vi "適應性控制_輸入權重係數模式(實際控制).vi"() -> ()   [LabVIEW 2010]
panel:
  in  "權重函數向量":dbl[](array[numeric])
  out "while平均時間(ms)":dbl
  out "當下ERR":dbl
  in  "number of samples":i32=100
  in  "rate":dbl=1000.0
  out "收斂時間(s)":dbl
  out "收斂燈":bool
  in  "ERR誤差低於多少V亮燈":dbl=0.05
  out "ERR message":string=" INSTRUCTIONS:\r\rNormal Use:  When using subVIs that incorporate the error in/error out (or error I/O) structure, place this handler where you want to inform the user of an error, typically at the end of the I/O data path, as the last action of the program.  If the error in error? is ERROR, the handler creates a message describing the error and its source.  If the type of dialog = 1 (default), the message is displayed to the user, who can only acknowedge it.  If the type = 2, the user can acknowledge the message or abort execution; aborting a program with active I/O is not recommended.  If the type = 0, no message is displayed; this is used to process the error programmatically, and the error out cluster elements are wired to individual terminals for that reason.  \r\rOther Use:\n\r\nlocal testing.  To test the error code of a subVI or function that does not have the error I/O structure, you can wire its error code and a source string to the local error code and error source inputs.  If error in error? indicates no error and error code is not equal to 0, the local code and source are substituted for the error in values, and error? is set TRUE (ERROR)."
  out "理想系統與FIR輸出":cluster{dbl, dbl, dbl}(graph)
  out "system輸出":dbl
  out "input_x(t)":dbl(graph)
  in  "order":i32=8
  out "FIR輸出":dbl
  in  "Stop Button":bool
  # "A0:模擬輸入 pulse_output 2"
  # "A1:理想系統 pulse_output 1"
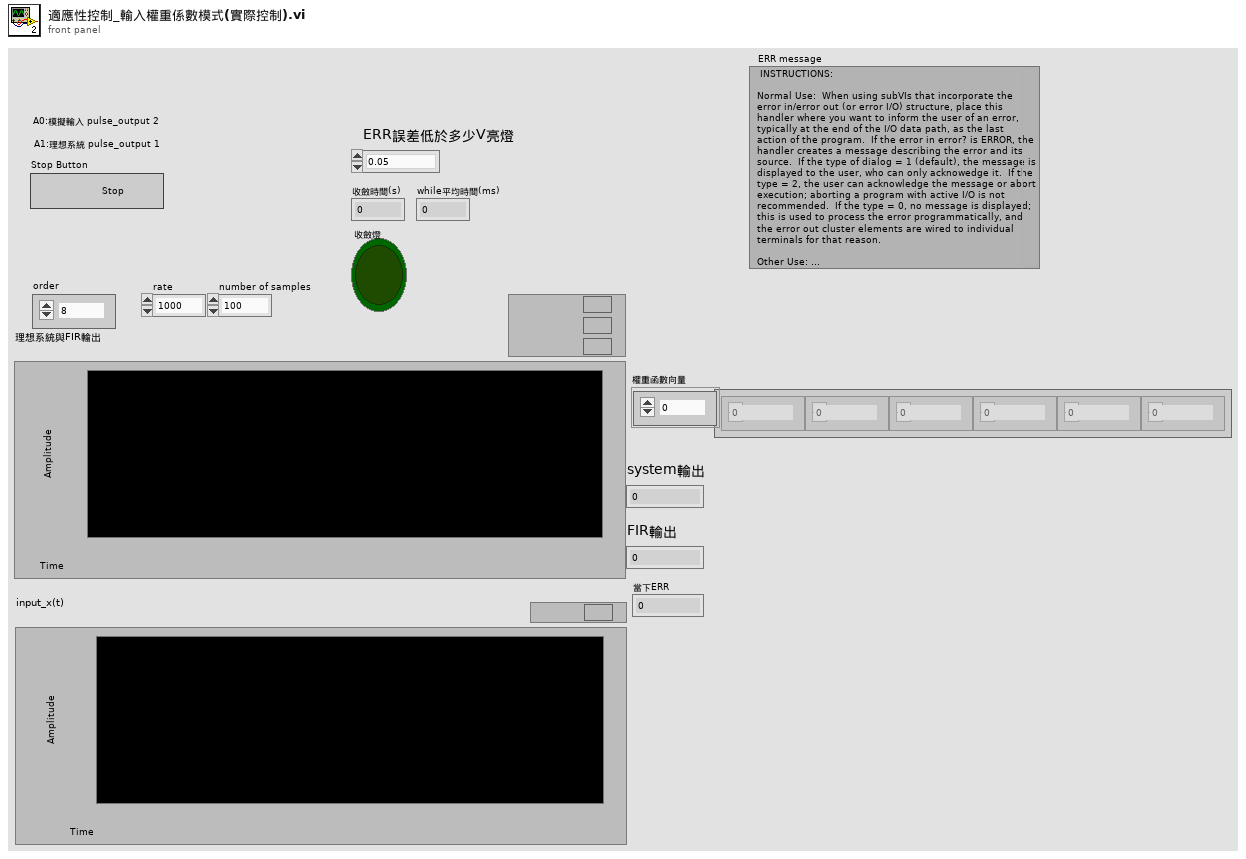
[diagram p1: front panel]
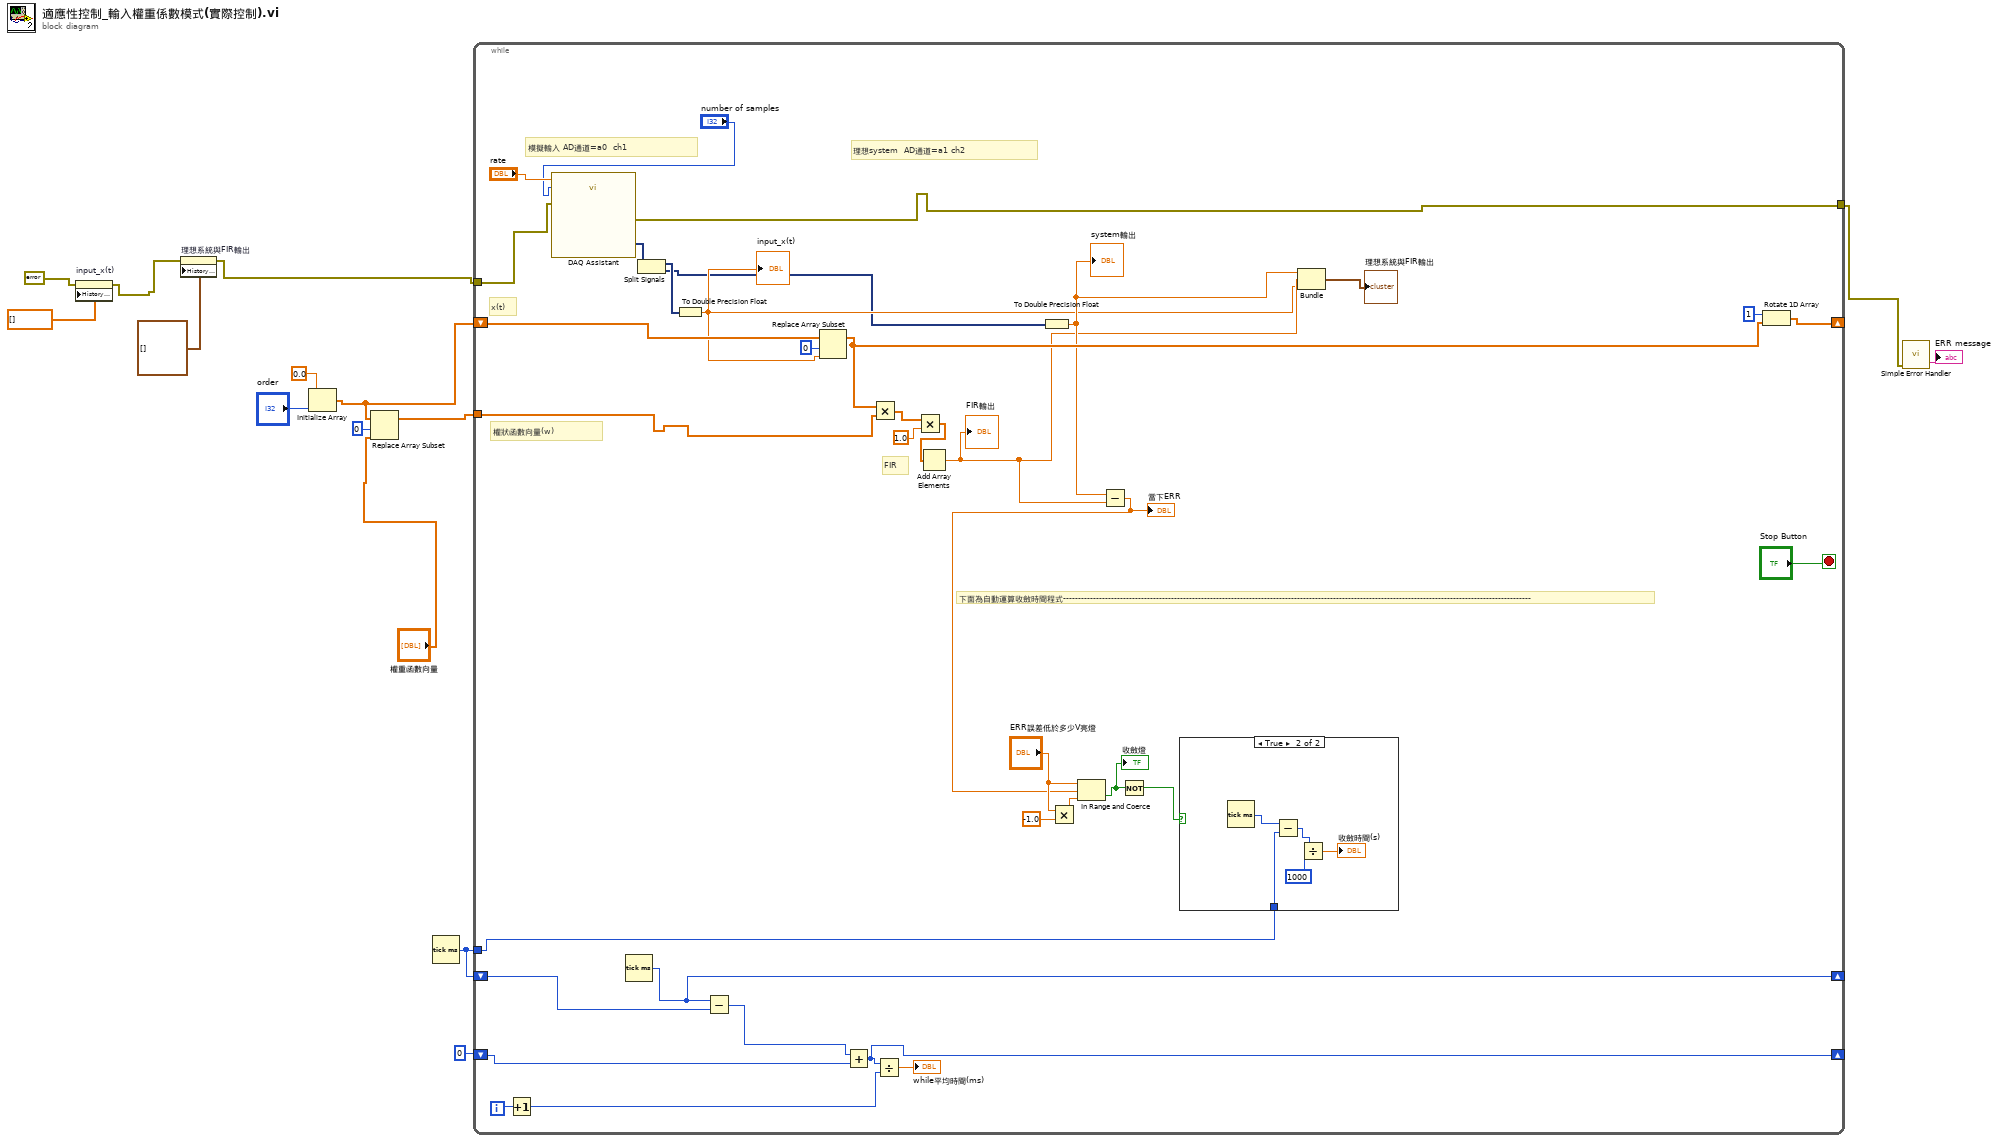
[diagram p0: block diagram]
diagram:
  n1 = property on="input_x(t)" class="WFChart (strict)"(error in=errorcluster {"status"=FALSE, "code"=0, "source"=""} ("error constant"), "History Data"=dbl[] []) -> (error out=w11:errorcluster)  [unwired: 1 in, 1 out]
  n2 = property on="理想系統與FIR輸出" class="WFChart (strict)"(error in=w11, "History Data"=cluster{dbl, dbl, dbl}[] []) -> (error out=w5:errorcluster)  [unwired: 1 in, 1 out]
  n3 = Initialize Array "Initialize Array"(0.0 ("element"), "order") -> (w7:dbl[])
  n4 = Replace Array Subset(array=w7, new element="權重函數向量", index=0) -> (w4:dbl[])
  n5 = Tick Count (ms)() -> (millisecond timer value=w8:u32)
  n6 = while {
    shift-right: [w46] -> _
    shift-left: w7 -> [w45]
    tunnel: w5 -> [w42]
    tunnel: [w17] -> w10
    shift-right: [w32] -> _
    shift-left: w8 -> [w34]
    tunnel: w8 -> [w33]
    tunnel: w4 -> [w16]
    shift-right: [w21] -> _
    shift-left: u32 0 ("y") -> [w26]
    i -> [w24]
    stop <- "Stop Button" stop-if-true
    # "下面為自動運算收斂時間程式------------------------------------------------------------------------------------------------------------------------------------------------------------"
    # "FIR"
    # "模擬輸入 AD通道=a0  ch1"
    # "權狀函數向量(w)"
    # "x(t)"
    # "理想system  AD通道=a1 ch2"
    n7 = Increment(x=w24) -> (x+1=w23:i32)
    n8 = call "DAQ Assistant"("rate"="rate", "number of samples"="number of samples", "error in"=w42) -> ("data"=w20:dynamicdata, "error out"=w17:errorcluster)  [unwired: 13 in, 2 out]
    n9 = Tick Count (ms)() -> (millisecond timer value=w32:u32)
    n10 = Split Signals(w20) -> (w19:dynamicdata, w18:dynamicdata)  [unwired: 2 in]
    n11 = To Double Precision Float(number=w19) -> (double precision float=w27:dbl)
    "input_x(t)" <- w27
    n12 = Subtract(x=w32, y=w34) -> (x-y=w25:u32)
    n13 = Replace Array Subset "Replace Array Subset"(array=w45, new element=w27, index=0) -> (w43:dbl[])
    n14 = Add(x=w25, y=w26) -> (x+y=w21:u32)
    n15 = Multiply(x=w43, y=w16) -> (x*y=w51:dbl[])
    n16 = Divide(x=w21, y=w23) -> (x/y=→"while平均時間(ms)":dbl)
    n17 = Multiply(x=w51, y=1.0) -> (x*y=w48:dbl[])
    n18 = Add Array Elements(numeric array=w48) -> (sum=w29:dbl)
    "FIR輸出" <- w29
    n19 = To Double Precision Float(number=w18) -> (double precision float=w30:dbl)
    "system輸出" <- w30
    n20 = Multiply(x="ERR誤差低於多少V亮燈", y=-1.0) -> (x*y=w40:dbl)
    n21 = Subtract(x=w30, y=w29) -> (x-y=w28:dbl)
    "當下ERR" <- w28
    n22 = In Range and Coerce(upper limit="ERR誤差低於多少V亮燈", x=w28, lower limit=w40) -> (In Range?=w36:bool)  [unwired: 1 out]
    "收斂燈" <- w36
    n23 = Not(x=w36) -> (.not. x?=w37:bool)
    n24 = case shown="True" w37 {
      tunnel: w33 -> [_ w55]
      frame False {
      }
      frame True {
        n25 = Tick Count (ms)() -> (millisecond timer value=w56:u32)
        n26 = Subtract(x=w56, y=w55) -> (x-y=w54:u32)
        n27 = Divide(x=w54, y=u32 1000) -> (x/y=→"收斂時間(s)":dbl)
      }
    }
    n28 = Bundle(w30, w29, w27) -> (→"理想系統與FIR輸出":cluster{dbl, dbl, dbl})  [unwired: 1 in]
    n29 = Rotate 1D Array(1:w43, 2:1 ("n")) -> (0:w46:dbl[])
  }
  n30 = call <vilib>:"Simple Error Handler.vi"("error in (no error)"=w10) -> ("message"=→"ERR message":string)  [unwired: 4 in, 4 out]
